vi "Test_WriteFloat_ReadCorrectValue.vi"(8 "error in (no error)":errorcluster, 11 "TestCase in":refnum<class "TestSQliteDatabaseConfiguration.lvclass">) -> (0 "error out":errorcluster, 3 "TestCase out":refnum<class "TestSQliteDatabaseConfiguration.lvclass">)   [LabVIEW 2020, in "SQlite cfg tests.lvlib" / "TestSQliteDatabaseConfiguration.lvclass"]
uses:
  TestSQliteDatabaseConfiguration.lvclass
  TestSQliteDatabaseConfiguration.lvclass/TestSQliteDatabaseConfiguration.ctl
  <vilib>/gpm_packages/@cs/Configuration/Source/ConfigurationReference/ConfigurationReference.lvclass/ConfigurationReference.ctl
  e002e558-d5e5-459d-ba9e-71d9a5a75879.vi
  1bb3110a-552d-4b56-8dd7-594c2a54aa03.vi
  <vilib>/gpm_packages/@cs/Configuration/Source/ConfigurationReference/Explain DVR Error.vi
  e002e558-d5e5-459d-ba9e-71d9a5a75879.vi/8402ebc0-384b-46ab-989c-700e41096983.vi
  <vilib>/gpm_packages/@cs/Configuration/Source/ConfigurationReference/Read IConfiguration.vi
  <vilib>/gpm_packages/@cs/Configuration/Source/ConfigurationReference/Write IConfiguration.vi
  1bb3110a-552d-4b56-8dd7-594c2a54aa03.vi/7595dcc0-0a31-43e1-86ad-579fe37a7e85.vi
  <vilib>/gpm_packages/@cs/Configuration/Source/IConfiguration/Write SGL.vi
  <vilib>/gpm_packages/@cs/Configuration/Source/IConfiguration/Read SGL.vi
  Source/sqlite-queries/sqlite-queries.lvclass
  D:/Project/Labview-Projects/database-configuration/Source/IConfigDBQueries/IConfigurationDatabaseQueries.lvclass
  Source/configuration-database.lvclass
  C:/Program Files/National Instruments/LabVIEW 2020/vi.lib/gpm_packages/@cs/Configuration/Source/IConfiguration/IConfiguration.lvclass
  <vilib>/gpm_packages/@cs/Configuration/Source/IConfiguration/IConfiguration.lvclass
  <vilib>/gpm_packages/@cs/Configuration/Source/ConfigurationReference/ConfigurationReference.lvclass
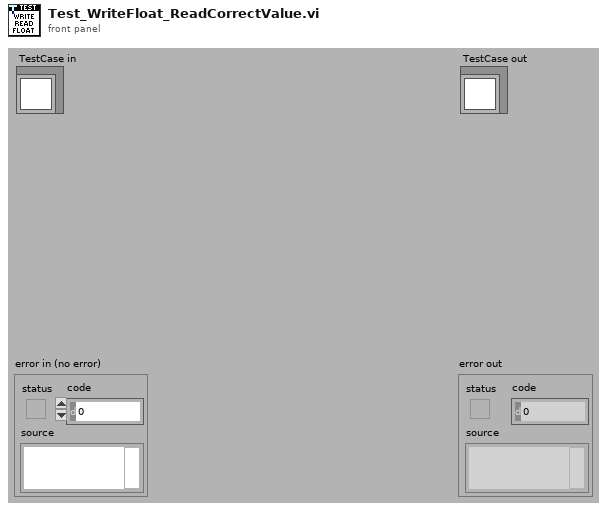
[diagram p1: front panel]
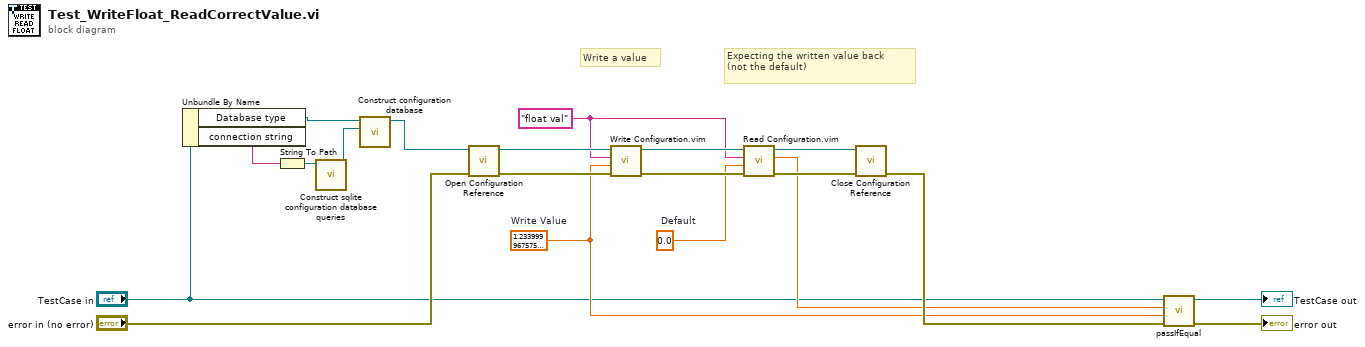
[diagram p0: block diagram]
diagram:
  w12 = sgl 0.0  # Default
  w7 = sgl 1.234  # Write Value
  w13 = "float val" ("Name")
  # "Write a value"
  # "Expecting the written value back\n(not the default)"
  n1 = Unbundle By Name("TestCase in") -> ("Database type"=w6:refnum<class "IDatabase.lvclass">, "connection string"=w2:string)
  n2 = String To Path(string=w2) -> (path=w3:path)
  n3 = call "Construct sqlite configuration database queries.vi"("database path"=w3) -> ("sqlite-configdb-queries out"=w1:refnum<class "sqlite-queries.lvclass">)  [unwired: 9 in, 1 out]
  n4 = call "Construct configuration database.vi"("SQL logic type"=w1, "Database type in"=w6) -> ("database-configuration out"=w5:refnum<class "configuration-database.lvclass">)  [unwired: 8 in, 1 out]
  n5 = call <vilib>:"Open Configuration Reference.vi"("error in (no error)"="error in (no error)", "Configuration Type"=w5) -> ("error out"=w14:errorcluster, "Configuration Reference"=w15:refnum<data-value>)  [unwired: 8 in]
  n6 = call "Write Configuration.vim"("error in (no error)"=w14, "Value"=w7, "Name"=w13, "Configuration Reference in"=w15) -> ("error out"=w16:errorcluster, "Configuration Reference out"=w17:refnum<data-value>)  [unwired: 6 in]
  n7 = call "Read Configuration.vim"("error in (no error)"=w16, "Type (Default Value If Not Found)"=w12, "Name"=w13, "Configuration Reference in"=w17) -> ("error out"=w10:errorcluster, "Value"=w8:sgl, "Configuration Reference out"=w11:refnum<data-value>)  [unwired: 4 in, 1 out]
  n8 = call <vilib>:"Close Configuration Reference.vi"("error in (no error)"=w10, "Configuration Reference"=w11) -> ("error out"=w9:errorcluster)  [unwired: 9 in]
  n9 = call-dynamic "passIfEqual.vi"("error in (no error)"=w9, "y"=w7, "x"=w8, "TestCase in"="TestCase in") -> ("error out"=→"error out":errorcluster, "TestCase out"=→"TestCase out":refnum<class "TestSQliteDatabaseConfiguration.lvclass">)  [unwired: 6 in]
